vi "Endpoint.vi"(6 "abort (F)":bool, 9 "element in":T2) -> (0 "missed":i32, 1 "element out":T2, 3 "channel out":T1, 4 "aborted?":bool)   [LabVIEW 2020]
uses:
  Flex.lvlib
  ChannelOp.ctl
  Element.ctl
  ))Channel.ctl
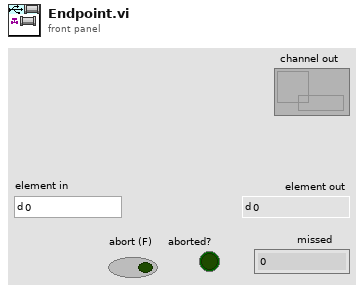
[diagram p1: front panel]
types:
  T1 = typedef "Flex.lvlib/))Channel.ctl" = refnum<queue>
  T2 = typedef "Flex.lvlib/Element.ctl" = dbl
  T3 = typedef "Flex.lvlib/ChannelOp.ctl" = enum16{"Init", "Close", "Probe", "New Queue"}
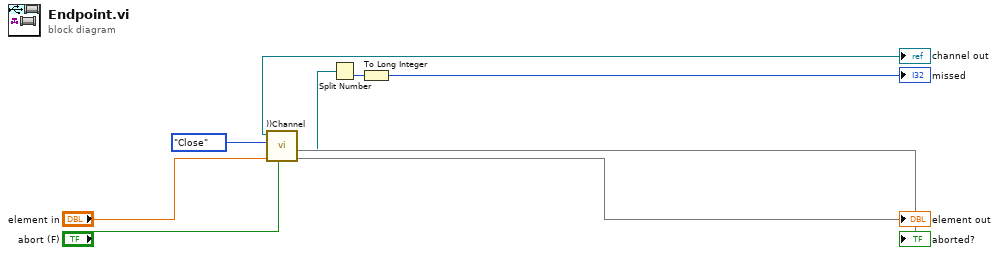
[diagram p0: block diagram]
diagram:
  n1 = call "))Channel.vi"(6:"abort (F)", 8:"element in", "channelOp"=ChannelOp."Close", "channel in"="channel out") -> (0:→"element out", "New Queue"=w3:refnum<queue>, 4:→"aborted?")  [unwired: 2 in, 3 out]
  n2 = Split Number(x=w3) -> (lo(x)=w1:u16)  [unwired: 1 out]
  n3 = To Long Integer(number=w1) -> (32bit integer=→"missed":i32)
